vi "create multi-color image U16(SubVI).vi"(6 "Zoom":sgl, 9 "Array":u16[][][](array[numeric]), 10 "Cluster":T1, 11 "Picture in":refnum<vi>) -> (3 "new picture 2":picture)   [LabVIEW 2024]
uses:
  <vilib>/Utility/miscctls.llb/LVBoundsTypeDef.ctl
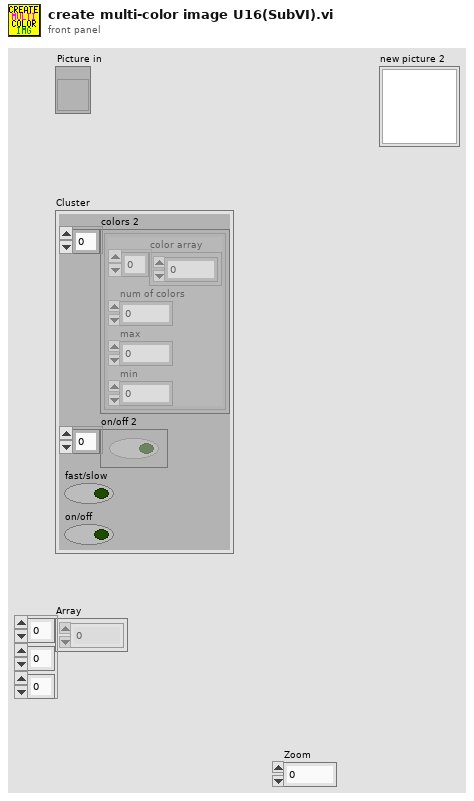
[diagram p1: front panel]
types:
  T1 = cluster{"colors 2":cluster{"color array":u32[], "num of colors":i32, "max":dbl, "min":dbl}[], "on/off 2":bool[], "fast/slow":bool, "on/off":bool}
  T2 = cluster{"color array":u32[], "num of colors":i32, "max":dbl, "min":dbl}[]
  T3 = typedef "LVBoundsTypeDef.ctl" = cluster{"Width":u32, "Height":u32}
  T4 = typedef "imagedata.ctl" = cluster{"image type":i32, "image depth":i32, "image":u8[], "mask":u8[], "colors":u32[], "Rectangle":cluster{"left":i16, "top":i16, "right":i16, "bottom":i16}}
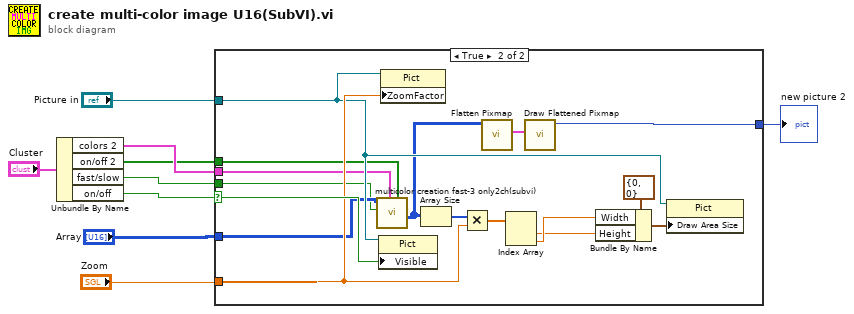
[diagram p0: block diagram]
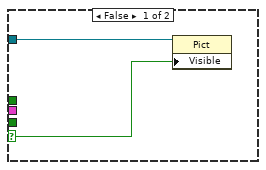
[diagram p2: hidden frame]
diagram:
  n1 = Unbundle By Name("Cluster") -> ("colors 2"=w8:T2, "on/off 2"=w6:bool[], "fast/slow"=w7:bool, "on/off"=w5:bool)
  n2 = case shown="True" w5 {
    selector: w5 -> [w11 w19]
    tunnel: [_ w20] -> w1
    tunnel: "Zoom" -> [_ w18]
    tunnel: "Picture in" -> [w10 w17]
    tunnel: w6 -> [_ w15]
    tunnel: w7 -> [_ w13]
    tunnel: w8 -> [_ w16]
    tunnel: "Array" -> [_ w14]
    frame False {
      n3 = property on="Property Node" class="Pict"(reference=w10, "Visible"=w11) -> ()  [unwired: 1 in, 2 out]
    }
    frame True {
      n4 = call "multicolor creation fast-3 only2ch(subvi).vi"("on/off"=w15, "colors"=w16, "fast/slow"=w13, "img array in"=w14) -> ("mixed img array"=w12:u32[][])  [unwired: 5 in]
      n5 = property on="Property Node" class="Pict"(reference=w17, "Visible"=w19) -> ()  [unwired: 1 in, 2 out]
      n6 = property on="Property Node" class="Pict"(reference=w17, "ZoomFactor"=w18) -> ()  [unwired: 1 in, 2 out]
      n7 = Array Size(array=w12) -> (size(s)=w25:i32[])
      n8 = Multiply(x=w25, y=w18) -> (x*y=w21:sgl[])
      n9 = call <vilib>:"Flatten Pixmap.vi"("24-bit pixmap"=w12) -> ("image data"=w27:T4)  [unwired: 10 in]
      n10 = Index Array(array=w21) -> (element #1=w23:sgl, element #2=w24:sgl)  [unwired: 2 in]
      n11 = call <vilib>:"Draw Flattened Pixmap.vi"("image data"=w27) -> ("new picture"=w20:picture)  [unwired: 8 in]
      n12 = Bundle By Name(cluster=T3 {"Width"=0, "Height"=0} ("Draw Area Size"), "Width"=w24, "Height"=w23) -> (w22:T3)
      n13 = property on="Property Node" class="Pict"(reference=w17, "Draw Area Size"=w22) -> ()  [unwired: 1 in, 2 out]
    }
  }
  "new picture 2" <- w1
